vi "Read Cooler ON_OFF.vi"(8 "error in (no error)":errorcluster, 11 "CCDCamera in":refnum<class "CCDCamera.lvclass">) -> (0 "error out":errorcluster, 2 "Cooler ON/OFF":u8, 3 "CCDCamera out":refnum<class "CCDCamera.lvclass">)   [LabVIEW 2018, in "CCDCamera.lvclass"]
uses:
  CCDCamera.lvclass
  CCDCamera.lvclass/CCDCamera.ctl
  Cooler/Cooler.lvclass/Cooler.ctl
  Cooler/Cooler.lvclass
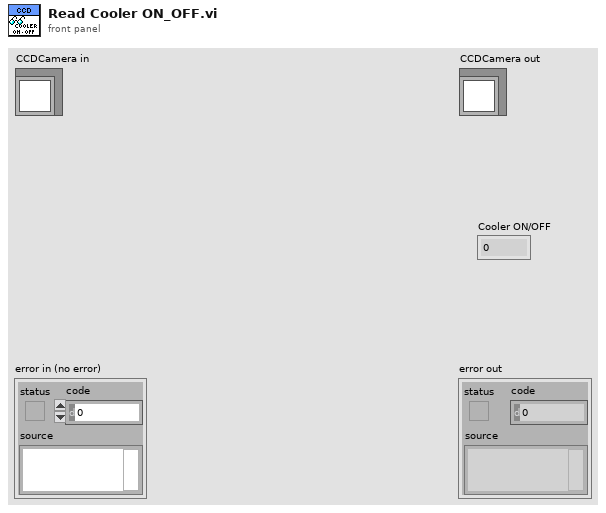
[diagram p1: front panel]
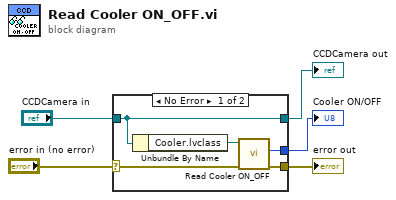
[diagram p0: block diagram]
diagram:
  n1 = case shown="No Error" "error in (no error)" {
    selector: "error in (no error)" -> [w8 w12]
    tunnel: [w9 w12] -> w4
    tunnel: [w10 w11] -> w2
    tunnel: "CCDCamera in" -> [w10 w11]
    tunnel: [w6 _] -> w1
    frame No Error {
      n2 = Unbundle By Name(w10) -> ("Cooler.lvclass"=w7:refnum<class "Cooler.lvclass">)
      n3 = call "Read Cooler ON_OFF.vi"("error in (no error)"=w8, "Cooler in"=w7) -> ("error out"=w9:errorcluster, "Cooler ON/OFF"=w6:u8)  [unwired: 7 in, 1 out]
    }
    frame Error {
    }
  }
  "error out" <- w4
  "CCDCamera out" <- w2
  "Cooler ON/OFF" <- w1
